vi "Do.vi"(8 "error in (no error)":errorcluster, 10 "Actor in":refnum<class "Actor.lvclass">, 11 "Calibrate Potentiometers Msg in":refnum<class "Calibrate Potentiometers Msg.lvclass">) -> (0 "error out":errorcluster, 2 "Actor out":refnum<class "Actor.lvclass">)   [LabVIEW 2020, in "NI Force Task.lvlib" / "Calibrate Potentiometers Msg.lvclass"]
doc: "(<B>Filename</B>: Actor Framework.lvlib:Message.lvclass:Do.vi)\n\nDefines what a message does when it is received by an actor. Generally, a message instructs an actor to invoke one of its methods. By default, this method does nothing. A child class must override it to define behavior. Create a child class by using the Actor Framework Message Maker dialog box."
uses:
  Calibrate Potentiometers Msg.lvclass
  <vilib>/ActorFramework/Actor/Actor.lvclass
  NI Force Task/NI Force Task.lvclass
  C:/Program Files/National Instruments/LabVIEW 2020/vi.lib/ActorFramework/Actor/Actor.lvclass
  Calibrate Potentiometers Msg.lvclass/Calibrate Potentiometers Msg.ctl
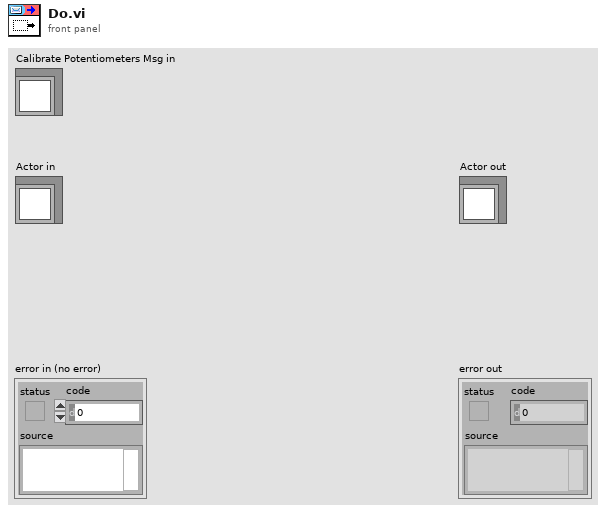
[diagram p1: front panel]
types:
  T1 = cluster{"Force Transducer: Left":tag, "Force Transducer: Right ":tag, "EMG: Left":tag, "EMG: Right":tag, "Potentiometer: Left":tag, "Potentiometer: Right":tag}
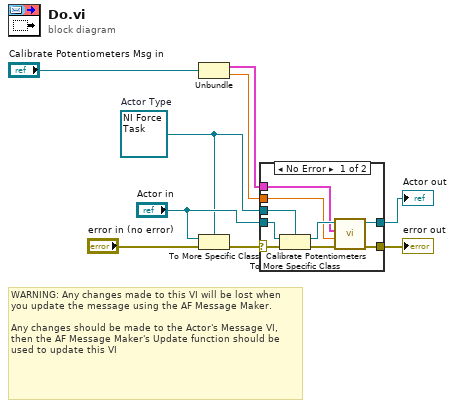
[diagram p0: block diagram]
diagram:
  w4 = refnum<class "NI Force Task.lvclass"> refnum  # Actor Type
  # "WARNING: Any changes made to this VI will be lost when you update the message using the AF Message Maker.\n\nAny changes should be made to the Actor's Message VI, then the AF Message Maker's Update function should be used to update this VI"
  n1 = Unbundle("Calibrate Potentiometers Msg in") -> (w3:T1, w2:dbl)
  n2 = To More Specific Class(target class=w4, reference="Actor in", error in="error in (no error)") -> (error out=w8:errorcluster)  [unwired: 1 out]
  n3 = case shown="No Error" w8 {
    selector: w8 -> [w18 w20]
    tunnel: [w13 w20] -> w7
    tunnel: [w12 w19] -> w6
    tunnel: "Actor in" -> [w17 w19]
    tunnel: w4 -> [w16 _]
    tunnel: w3 -> [w11 _]
    tunnel: w2 -> [w10 _]
    frame No Error {
      n4 = To More Specific Class ("Actor Cast")(target class=w16, reference=w17, error in=w18) -> (specific class reference=w15:refnum<class "NI Force Task.lvclass">, error out=w14:errorcluster)
      n5 = call "Calibrate Potentiometers.vi"("error in (no error)"=w14, "rate"=w10, "DAQ  Channels In"=w11, "NI Force Task in"=w15) -> ("error out"=w13:errorcluster, "NI Force Task out"=w12:refnum<class "NI Force Task.lvclass">)  [unwired: 6 in]
    }
    frame Error {
    }
  }
  "error out" <- w7
  "Actor out" <- w6
